vi "Store Configuration Parameters.vi"(8 "error in (no error)":errorcluster, 10 "refnum":T1, 11 "Example Configuration Dialog in":refnum<class "LogicIO Configuration.lvclass">) -> (0 "error out":errorcluster, 2 "refnum out":T1, 3 "Example Configuration Dialog out":refnum<class "LogicIO Configuration.lvclass">)   [LabVIEW 2016, in "Hardware.lvlib" / "LogicIO.lvlib" / "LogicIO Configuration.lvclass"]
uses:
  <userlib>/Common Components/Hardware/LogicIO/LogicIO Config/LogicIO Configuration.lvclass
  <vilib>/Utility/config.llb/Config Data RefNum.ctl
  <userlib>/Common Components/Hardware/LogicIO/LogicIO Config/LogicIO Configuration.lvclass/LogicIO Configuration.ctl
  <userlib>/Common Components/Hardware/Abstract Hardware/Hardware.lvclass/Hardware.ctl
  <userlib>/Common Components/Hardware/DevInfo/DevInfo.lvclass/DevInfo.ctl
  <userlib>/Common Components/Hardware/Abstract Hardware/Read Label.vi
  <userlib>/Common Components/Hardware/Abstract Hardware/Read DevInfo.vi
  <userlib>/Common Components/Hardware/DevInfo/Read HW Type.vi
  <userlib>/Common Components/Hardware/DevInfo/Read Device Name.vi
  <userlib>/Common Components/Hardware/DevInfo/Read COMM Address.vi
  <userlib>/Common Components/Hardware/DevInfo/Read Sub-COMM Address.vi
  <userlib>/Common Components/Hardware/LogicIO/LogicIO/LogicIO.lvclass
  C:/Program Files (x86)/National Instruments/LabVIEW 2016/user.lib/Common Components/Hardware/Abstract Hardware/Hardware.lvclass
  <userlib>/Common Components/Hardware/DevInfo/DevInfo.lvclass
  <vilib>/Utility/config.llb/NI_LVConfig.lvlib
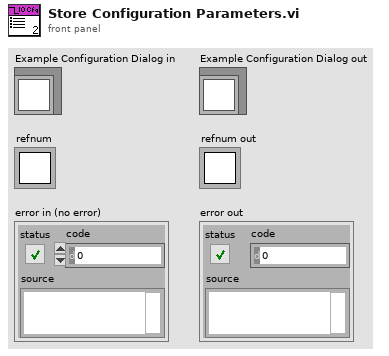
[diagram p1: front panel]
types:
  T1 = typedef "NI_LVConfig.lvlib/Config Data RefNum.ctl" = refnum<k1>
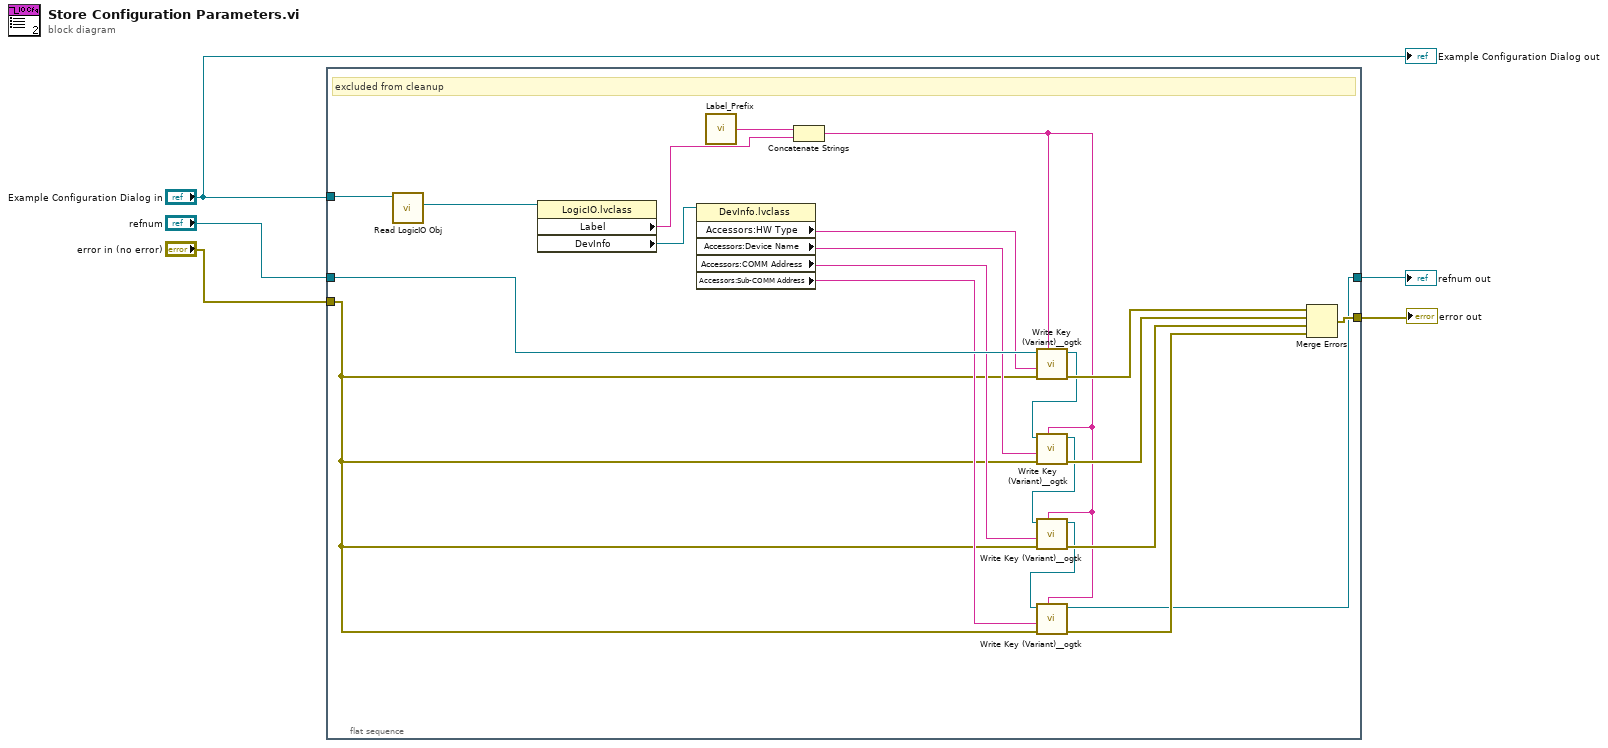
[diagram p0: block diagram]
diagram:
  n1 = flat-sequence {
    tunnel: "refnum" -> [w26]
    tunnel: "error in (no error)" -> [w6]
    tunnel: "Example Configuration Dialog in" -> [w25]
    tunnel: [w8] -> w2
    tunnel: [w24] -> w1
    frame #0 {
      # "excluded from cleanup"
      n2 = call <userlib>:"Read LogicIO Obj.vi"("LogicIO Configuration in"=w25) -> ("Hardware.lvlib:LogicIO.lvlib:LogicIO.lvclass"=w9:refnum<class "LogicIO.lvclass">)  [unwired: 9 in, 1 out]
      n3 = property class="LogicIO.lvclass"(reference=w9) -> ("Label"=w15:string, "DevInfo"=w14:refnum<class "DevInfo.lvclass">)  [unwired: 1 in, 2 out]
      n4 = property class="DevInfo.lvclass"(reference=w14) -> ("Accessors:HW Type"=w13:string, "Accessors:Device Name"=w12:string, "Accessors:COMM Address"=w11:string, "Accessors:Sub-COMM Address"=w10:string)  [unwired: 1 in, 2 out]
      n5 = call <userlib>:"Label_Prefix.vi"() -> ("Label Prefix String"=w23:string)
      n6 = Concatenate Strings(w23, w15) -> (w7:string)
      n7 = call <userlib>:"Write Key (Variant)__ogtk.vi"("section"=w7, "error in (no error)"=w6, "key-value"=w13, "refnum"=w26) -> ("error out"=w22:errorcluster, "refnum out"=w18:T1)  [unwired: 6 in]
      n8 = call <userlib>:"Write Key (Variant)__ogtk.vi"("section"=w7, "error in (no error)"=w6, "key-value"=w12, "refnum"=w18) -> ("error out"=w21:errorcluster, "refnum out"=w17:T1)  [unwired: 6 in]
      n9 = call <userlib>:"Write Key (Variant)__ogtk.vi"("section"=w7, "error in (no error)"=w6, "key-value"=w11, "refnum"=w17) -> ("error out"=w20:errorcluster, "refnum out"=w16:T1)  [unwired: 6 in]
      n10 = call <userlib>:"Write Key (Variant)__ogtk.vi"("section"=w7, "error in (no error)"=w6, "key-value"=w10, "refnum"=w16) -> ("error out"=w19:errorcluster, "refnum out"=w8:T1)  [unwired: 6 in]
      n11 = Merge Errors(w22, w21, w20, w19) -> (w24:errorcluster)
    }
  }
  "Example Configuration Dialog out" <- "Example Configuration Dialog in"
  "error out" <- w1
  "refnum out" <- w2
